vi "UDP volume send (subVI).vi"(5 "timestamp":dbl, 6 "Packet size":i32=65507, 7 "local port":u16=61556, 8 "error in (no error)":errorcluster, 9 "port of receiver":u16=61557, 10 "address":string="localhost", 11 "frame data":u16[][](array[numeric])) -> (0 "error out":errorcluster)   [LabVIEW 2024]
panel:
  out "Time(ms) 3":dbl
  out "Time1(ms)":dbl
  out "Packets":i32
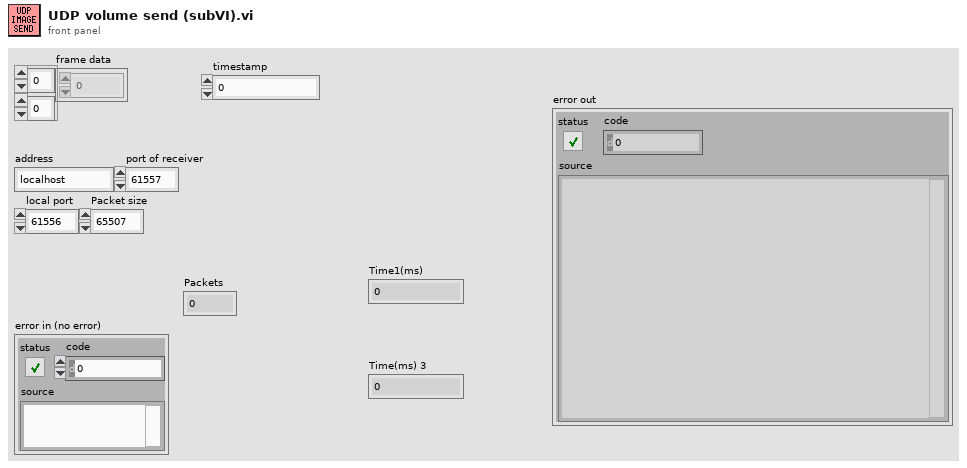
[diagram p1: front panel]
types:
  T1 = enum16{"big-endian, network order", "native, host order", "little-endian"}
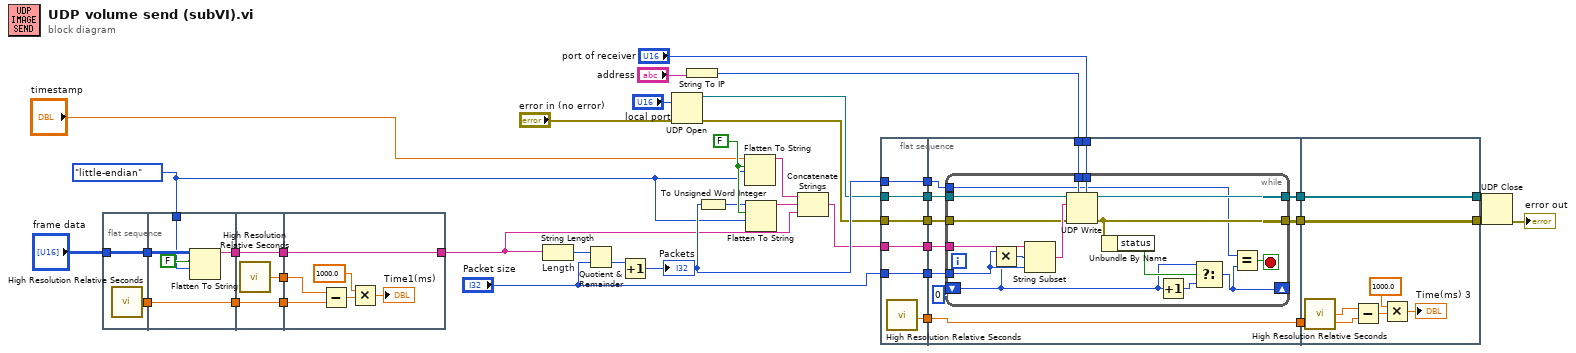
[diagram p0: block diagram]
diagram:
  w4 = T1."little-endian" ("byte order (0:big-endian, network order)")
  w6 = FALSE ("prepend array or string size? (T)")
  n1 = flat-sequence {
    tunnel: "frame data" -> [w41]
    tunnel: [w41] -> w33
    tunnel: [w40] -> w32
    tunnel: [w45] -> w31
    tunnel: w33 -> [w46]
    tunnel: [w43] -> w30
    tunnel: w32 -> [w43]
    tunnel: w4 -> [w42]
    tunnel: w31 -> [w49]
    tunnel: [w49] -> w29
    tunnel: [w48] -> w28
    tunnel: [w47] -> w27
    tunnel: w30 -> [w47]
    tunnel: [w55] -> w5
    tunnel: w29 -> [w55]
    tunnel: w28 -> [w51]
    tunnel: w27 -> [w50]
    frame #0 {
      n2 = call <vilib>:"High Resolution Relative Seconds.vi"() -> ("relative seconds"=w40:dbl)
    }
    frame #1 {
      n3 = Flatten To String(anything=w46, prepend array or string size? (T)=FALSE, byte order (0:big-endian, network order)=w42) -> (data string=w45:string)  [unwired: 1 in, 2 out]
    }
    frame #2 {
      n4 = call <vilib>:"High Resolution Relative Seconds.vi"() -> ("relative seconds"=w48:dbl)
    }
    frame #3 {
      n5 = Subtract(x=w51, y=w50) -> (x-y=w53:dbl)
      n6 = Multiply(x=1000.0, y=w53) -> (x*y=→"Time1(ms)":dbl)
    }
  }
  n7 = String Length "Length"(string=w5) -> (length=w12:i32)
  n8 = Quotient & Remainder(x=w12, y="Packet size") -> (floor(x/y)=w13:i32)  [unwired: 1 out]
  n9 = Increment(x=w13) -> (x+1=w26:i32)
  "Packets" <- w26
  n10 = UDP Open(8:"error in (no error)", 11:"local port") -> (port=w8:refnum<k16>, 0:w7:errorcluster)  [unwired: 3 in, 1 out]
  n11 = String To IP(1:"address") -> (0:w34:u32)
  n12 = To Unsigned Word Integer(number=w26) -> (unsigned 16bit integer=w3:u16)
  n13 = Flatten To String(anything="timestamp", prepend array or string size? (T)=w6, byte order (0:big-endian, network order)=w4) -> (data string=w10:string)  [unwired: 1 in, 2 out]
  n14 = Flatten To String(anything=w3, prepend array or string size? (T)=w6, byte order (0:big-endian, network order)=w4) -> (data string=w11:string)  [unwired: 1 in, 2 out]
  n15 = Concatenate Strings(w10, w11, w5) -> (w9:string)
  n16 = flat-sequence {
    tunnel: w9 -> [w57]
    tunnel: "Packet size" -> [w58]
    tunnel: w26 -> [w59]
    tunnel: w7 -> [w60]
    tunnel: w8 -> [w61]
    tunnel: [w61] -> w20
    tunnel: [w60] -> w19
    tunnel: [w59] -> w18
    tunnel: [w58] -> w17
    tunnel: [w57] -> w16
    tunnel: [w56] -> w15
    tunnel: "port of receiver" -> [w70]
    tunnel: w34 -> [w69]
    tunnel: [w72] -> w22
    tunnel: [w71] -> w21
    tunnel: w20 -> [w68]
    tunnel: w19 -> [w67]
    tunnel: w18 -> [w62]
    tunnel: w17 -> [w66]
    tunnel: w16 -> [w65]
    tunnel: w15 -> [w64]
    tunnel: [w64] -> w14
    tunnel: [w94] -> w38
    tunnel: [w95] -> w39
    tunnel: w22 -> [w95]
    tunnel: w21 -> [w94]
    tunnel: w14 -> [w89]
    frame #0 {
      n17 = call <vilib>:"High Resolution Relative Seconds.vi"() -> ("relative seconds"=w56:dbl)
    }
    frame #1 {
      n18 = while {
        tunnel: w68 -> [w86]
        tunnel: w67 -> [w85]
        tunnel: w66 -> [w88]
        tunnel: [w79] -> w71
        tunnel: [w84] -> w72
        tunnel: w70 -> [w82]
        tunnel: w69 -> [w81]
        tunnel: w65 -> [w80]
        shift-right: [w74] -> _
        shift-left: 0 -> [w73]
        tunnel: w62 -> [w77]
        stop <- w78 stop-if-true
        n19 = Multiply(x=w88, y=w73) -> (x*y=w83:i32)
        n20 = String Subset(string=w80, offset (0)=w83, length (rest)=w88) -> (substring=w87:string)
        n21 = UDP Write(address=w81, port or service name=w82, connection ID=w86, data in=w87, 8:w85) -> (error out=w79:errorcluster, 3:w84:refnum<k16>)  [unwired: 1 in]
        n22 = Unbundle By Name(w79) -> ("status"=w76:bool)
        n23 = Increment(x=w73) -> (x+1=w75:i32)
        n24 = Select(t=w73, s=w76, f=w75) -> (s? t:f=w74:i32)
        n25 = Equal?(x=w77, y=w74) -> (x = y?=w78:bool)
      }
    }
    frame #2 {
      n26 = call <vilib>:"High Resolution Relative Seconds.vi"() -> ("relative seconds"=w90:dbl)
      n27 = Subtract(x=w90, y=w89) -> (x-y=w91:dbl)
      n28 = Multiply(x=1000.0, y=w91) -> (x*y=→"Time(ms) 3":dbl)
    }
  }
  n29 = UDP Close(connection ID=w39, 8:w38) -> (error out=→"error out":errorcluster)  [unwired: 1 out]
